vi "acq.Luminescence.vi"(5 "Delay":u16, 6 "mode":T1, 7 "DVR":T3, 8 "error in":errorcluster, 9 "# Acq in":i32, 10 "image":refnum<queue>) -> (0 "error out":errorcluster, 2 "Image Out":T2)   [LabVIEW 2020]
uses:
  6ca06af8-5255-4aa7-8013-97f442914d80.vi
  _controls/mode.ctl
  camera/camera.lvclass
  _controls/data.ref.ctl
  _controls/data.ctl
  _controls/state.ctl
  _controls/data.vars.ctl
  _controls/flip.ctl
  <vilib>/vision/Image Controls.llb/IMAQ Image.ctl
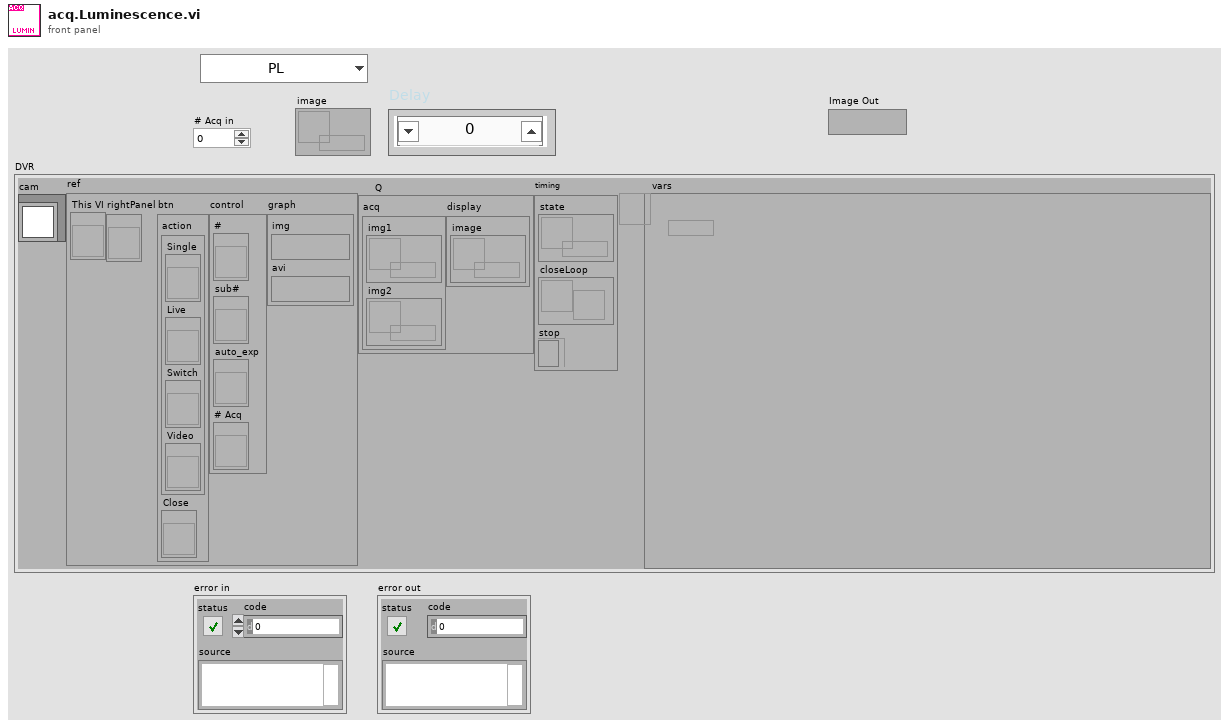
[diagram p1: front panel]
types:
  T1 = typedef "mode.ctl" = enum16{"PL", "EL"}
  T2 = typedef "IMAQ Image.ctl" = refnum<image>
  T3 = typedef "data.ctl" = cluster{"cam":refnum<class "camera.lvclass">, "ref":T4, "Q":cluster{"acq":cluster{"img1":refnum<queue>, "img2":refnum<queue>}, "display":cluster{"image":refnum<queue>}}, "timing":cluster{"state":refnum<queue>, "closeLoop":refnum<notifier>, "stop":refnum<k4>}, "vars":refnum<data-value>}
  T4 = typedef "data.ref.ctl" = cluster{"This VI":refnum<vi>, "rightPanel":refnum<vi>, "btn":cluster{"action":cluster{"Single":refnum<vi>, "Live":refnum<vi>, "Switch":refnum<vi>, "Video":refnum<vi>}, "Close":refnum<vi>}, "control":cluster{"#":refnum<vi>, "sub#":refnum<vi>, "auto_exp":refnum<vi>, "# Acq":refnum<vi>}, "graph":cluster{"img":T2, "avi":T2}}
  T5 = cluster{"img1":refnum<queue>, "img2":refnum<queue>}
  T6 = typedef "path.ctl" = cluster{"light":path, "name":string, "full":path}
  T7 = typedef "data.vars.ctl" = cluster{"save":cluster{"base_folder":cluster{"Folder":path, "tif":bool, "jpg":bool}, "module":string, "#":u32, "sub#":u8, "save.op":enum16{"Full", "Light"}, "same?":bool, "Shift":enum16{"Single", "Leapfrog"}, "jpg?":bool, "flip":T8}, "acq":cluster{"# Acq":u16, "rotate":bool, "FPS":dbl}, "calib.manual":cluster{"BG":cluster{"Image":u16[][], "enabled?":bool}, "FF":cluster{"Image":u16[][], "enabled?":bool}}}
  T8 = typedef "flip.ctl" = cluster{"x":bool, "y":bool}
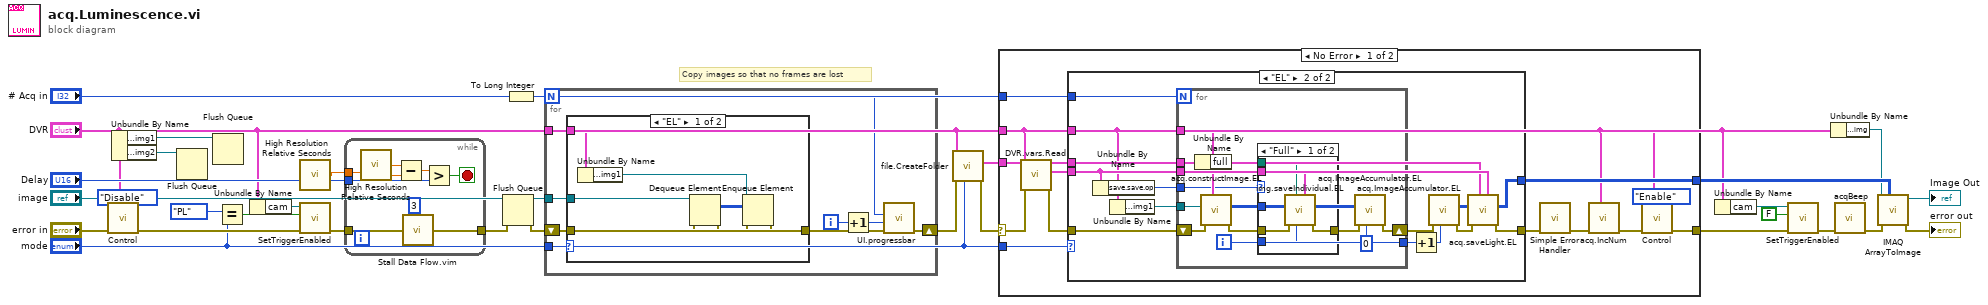
[diagram p0: block diagram]
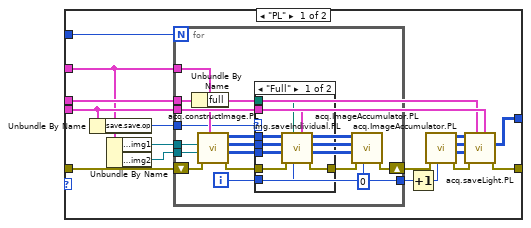
[diagram p2: hidden frame]
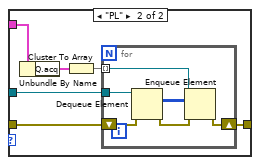
[diagram p6: hidden frame]
diagram:
  # "Copy images so that no frames are lost"
  n1 = call "Control.vi"("mode"=enum16{"Enable", "Disable"}."Disable", "DVR"="DVR", "error in"="error in") -> ("error out"=w17:errorcluster)  [unwired: 8 in]
  n2 = Unbundle By Name("DVR") -> ("Q.acq.img1"=w5:refnum<queue>, "Q.acq.img2"=w6:refnum<queue>)
  n3 = Flush Queue(queue=w6) -> ()  [unwired: 1 in, 3 out]
  n4 = Flush Queue(queue=w5) -> ()  [unwired: 1 in, 3 out]
  n5 = Equal?(x=mode."PL", y="mode") -> (x = y?=w8:bool)
  n6 = Unbundle By Name("DVR") -> ("cam"=w3:refnum<class "camera.lvclass">)
  n7 = call <vilib>:"High Resolution Relative Seconds.vi"() -> ("relative seconds"=w21:dbl)
  n8 = call "SetTriggerEnabled.vi"("error in"=w17, "trigger"=w8, "camera.nit in"=w3) -> ("error out"=w16:errorcluster)  [unwired: 8 in]
  n9 = while {
    tunnel: w21 -> [w37]
    tunnel: "Delay" -> [w35]
    tunnel: [w32] -> w11
    tunnel: w16 -> [w33]
    stop <- w34 stop-if-true
    n10 = call <vilib>:"High Resolution Relative Seconds.vi"() -> ("relative seconds"=w38:dbl)
    n11 = Subtract(x=w38, y=w37) -> (x-y=w36:dbl)
    n12 = call "Stall Data Flow.vim"("value in"=w33, "milliseconds to wait"=u32 3) -> ("value out"=w32:errorcluster)  [unwired: 1 out]
    n13 = Greater?(x=w36, y=w35) -> (0:w34:bool)
  }
  n14 = Flush Queue(queue="image", error in (no error)=w11) -> (queue out=w12:refnum<queue>, error out=w10:errorcluster)  [unwired: 1 out]
  n15 = To Long Integer(number="# Acq in") -> (32bit integer=w23:i32)
  n16 = for {
    N: w23 -> [w43]
    tunnel: w12 -> [w46]
    shift-right: [w42] -> _
    shift-left: w10 -> [w47]
    tunnel: "mode" -> [w40]
    tunnel: "DVR" -> [w39]
    i -> [w44]
    n17 = case shown="\"EL\"" w40 {
      tunnel: w47 -> [w54 w60]
      tunnel: w46 -> [w53 w59]
      tunnel: [w52 w58] -> w45
      tunnel: w39 -> [w49 w56]
      frame "EL" {
        n18 = Unbundle By Name(w49) -> ("Q.acq.img1"=w48:refnum<queue>)
        n19 = Dequeue Element(queue=w53, error in (no error)=w54) -> (element=w51:u16[][], error out=w50:errorcluster)  [unwired: 1 in, 2 out]
        n20 = Enqueue Element(queue=w48, element=w51, error in (no error)=w50) -> (error out=w52:errorcluster)  [unwired: 1 in, 2 out]
      }
      frame "PL" {
        n21 = Unbundle By Name(w56) -> ("Q.acq"=w57:T5)
        n22 = Cluster To Array(cluster=w57) -> (array=w55:refnum<queue>[])
        n23 = for {
          tunnel: w59 -> [w66]
          tunnel: w55 -> [w65] mode=indexing
          shift-right: [w62] -> w58
          shift-left: w60 -> [w61]
          n24 = Dequeue Element(queue=w66, error in (no error)=w61) -> (element=w64:u16[][], error out=w63:errorcluster)  [unwired: 1 in, 2 out]
          n25 = Enqueue Element(queue=w65, element=w64, error in (no error)=w63) -> (error out=w62:errorcluster)  [unwired: 1 in, 2 out]
        }
      }
    }
    n26 = Increment(x=w44) -> (x+1=w41:i32)
    n27 = call "UI.progressbar.vi"("error in"=w45, "Value"=w41, "Maximum"=w43) -> ("error out"=w42:errorcluster)  [unwired: 8 in]
  }
  n28 = call "file.CreateFolder.vi"("mode"="mode", "error in"=w10, "DVR"="DVR") -> ("error out"=w30:errorcluster, "path"=w29:T6)  [unwired: 7 in]
  n29 = case shown="No Error" w30 {
    selector: w30 -> [w69 w156]
    tunnel: w23 -> [w79 _]
    tunnel: "DVR" -> [w71 _]
    tunnel: [w76 w156] -> w15
    tunnel: [w73 _] -> w28
    tunnel: w29 -> [w72 _]
    tunnel: "mode" -> [w68 _]
    frame No Error {
      n30 = call "DVR.vars.Read.vi"("error in"=w69, "DVR.state"=w71) -> ("error out"=w78:errorcluster, "vars"=w74:T7)  [unwired: 8 in]
      n31 = case shown="\"EL\"" w68 {
        tunnel: w79 -> [w96 w135]
        tunnel: w78 -> [w95 w134]
        tunnel: [w94 w133] -> w75
        tunnel: w74 -> [w93 w132]
        tunnel: [w92 w131] -> w73
        tunnel: w72 -> [w90 w129]
        tunnel: w71 -> [w83 w124]
        frame "PL" {
          n32 = Unbundle By Name(w93) -> ("save.save.op"=w91:enum16{"Full", "Light"})
          n33 = Unbundle By Name(w83) -> ("Q.acq.img1"=w82:refnum<queue>, "Q.acq.img2"=w81:refnum<queue>)
          n34 = for {
            N: w96 -> [_]
            shift-right: [w99] -> w80
            shift-left: w95 -> [w109]
            tunnel: w90 -> [w112]
            tunnel: w81 -> [w110]
            tunnel: w82 -> [w111]
            tunnel: w83 -> [w108]
            tunnel: w93 -> [w106]
            tunnel: w91 -> [w105]
            tunnel: [w98] -> w85
            i -> [w98]
            n35 = Unbundle By Name(w112) -> ("full"=w104:path)
            n36 = call "acq.constructImage.PL.vi"("DVR"=w108, "error in"=w109, "queue2 in"=w110, "queue1 in"=w111) -> ("error out"=w107:errorcluster, "Dark"=w101:u16[][], "PL"=w102:u16[][], "Bright"=w103:u16[][])  [unwired: 4 in]
            n37 = case shown="\"Full\"" w105 {
              tunnel: w104 -> [w120 _]
              tunnel: w107 -> [w119 w121]
              tunnel: w98 -> [w113 _]
              tunnel: w103 -> [w118 _]
              tunnel: w102 -> [w117 _]
              tunnel: w106 -> [w116 _]
              tunnel: w101 -> [w115 _]
              tunnel: [w114 w121] -> w100
              frame "Full" {
                n38 = call "img.saveIndividual.PL.vi"("vars"=w116, "loop"=w113, "path"=w120, "error in"=w119, "Dark"=w115, "PL"=w117, "Bright"=w118) -> ("error out"=w114:errorcluster)  [unwired: 4 in]
              }
              frame "Light" {
              }
            }
            n39 = call "acq.ImageAccumulator.PL.vi"("loop"=0, "error in"=w100, "Dark in"=w101, "PL in"=w102, "Bright in"=w103) -> ("error out"=w99:errorcluster)  [unwired: 3 in, 3 out]
          }
          n40 = Increment(x=w85) -> (x+1=w84:i32)
          n41 = call "acq.ImageAccumulator.PL.vi"("loop"=w84, "error in"=w80) -> ("error out"=w89:errorcluster, "Dark out"=w88:u16[][], "PL out"=w87:u16[][], "Bright out"=w86:u16[][])  [unwired: 6 in]
          n42 = call "acq.saveLight.PL.vi"("vars"=w93, "path"=w90, "error in"=w89, "Dark"=w88, "PL"=w87, "Bright"=w86) -> ("error out"=w94:errorcluster, "PL"=w92:u16[][])  [unwired: 3 in, 1 out]
        }
        frame "EL" {
          n43 = Unbundle By Name(w132) -> ("save.save.op"=w130:enum16{"Full", "Light"})
          n44 = Unbundle By Name(w124) -> ("Q.acq.img1"=w123:refnum<queue>)
          n45 = for {
            N: w135 -> [_]
            shift-right: [w138] -> w122
            shift-left: w134 -> [w146]
            tunnel: w129 -> [w148]
            tunnel: w123 -> [w147]
            tunnel: w124 -> [w145]
            tunnel: w132 -> [w143]
            tunnel: w130 -> [w142]
            tunnel: [w137] -> w126
            i -> [w137]
            n46 = Unbundle By Name(w148) -> ("full"=w141:path)
            n47 = call "acq.constructImage.EL.vi"("DVR"=w145, "error in"=w146, "queue1 in"=w147) -> ("error out"=w144:errorcluster, "EL"=w140:u16[][])  [unwired: 7 in]
            n48 = case shown="\"Full\"" w142 {
              tunnel: w141 -> [w154 _]
              tunnel: w144 -> [w153 w155]
              tunnel: w137 -> [w149 _]
              tunnel: w140 -> [w152 _]
              tunnel: w143 -> [w151 _]
              tunnel: [w150 w155] -> w139
              frame "Full" {
                n49 = call "img.saveIndividual.EL.vi"("vars"=w151, "loop"=w149, "path"=w154, "error in"=w153, "EL"=w152) -> ("error out"=w150:errorcluster)  [unwired: 6 in]
              }
              frame "Light" {
              }
            }
            n50 = call "acq.ImageAccumulator.EL.vi"("loop"=0, "error in"=w139, "EL in"=w140) -> ("error out"=w138:errorcluster)  [unwired: 7 in, 1 out]
          }
          n51 = Increment(x=w126) -> (x+1=w125:i32)
          n52 = call "acq.ImageAccumulator.EL.vi"("loop"=w125, "error in"=w122) -> ("error out"=w128:errorcluster, "EL out"=w127:u16[][])  [unwired: 8 in]
          n53 = call "acq.saveLight.EL.vi"("vars"=w132, "path"=w129, "error in"=w128, "EL"=w127) -> ("error out"=w133:errorcluster, "EL"=w131:u16[][])  [unwired: 6 in]
        }
      }
      n54 = call <vilib>:"Simple Error Handler.vi"("error in (no error)"=w75) -> ("error out"=w67:errorcluster)  [unwired: 4 in, 4 out]
      n55 = call "acq.IncNum.vi"("DVR in"=w71, "error in"=w67) -> ("error out"=w70:errorcluster)  [unwired: 9 in]
      n56 = call "Control.vi"("mode"=enum16{"Enable", "Disable"}."Enable", "DVR"=w71, "error in"=w70) -> ("error out"=w76:errorcluster)  [unwired: 8 in]
    }
    frame Error {
    }
  }
  n57 = Unbundle By Name("DVR") -> ("cam"=w1:refnum<class "camera.lvclass">)
  n58 = call "SetTriggerEnabled.vi"("error in"=w15, "trigger"=FALSE, "camera.nit in"=w1) -> ("error out"=w14:errorcluster)  [unwired: 8 in]
  n59 = Unbundle By Name("DVR") -> ("ref.graph.img"=w25:T2)
  n60 = call "acqBeep.vi"("error in"=w14) -> ("error out"=w13:errorcluster)  [unwired: 10 in]
  n61 = call "IMAQ ArrayToImage"("Image Pixels (U16)"=w28, "error in (no error)"=w13, "Image"=w25) -> ("error out"=→"error out":errorcluster, "Image Out"=→"Image Out":T2)  [unwired: 7 in]
